vi "GetErrorLog.vi"(6 "Delay between send and receive [ms]":i32=100, 8 "error in (no error)":errorcluster, 11 "SCD in":refnum<class "SCD.lvclass">) -> (0 "error out":errorcluster, 1 "Found?":bool, 2 "errors":string[](array[string]), 3 "SCD out":refnum<class "SCD.lvclass">)   [LabVIEW 2023, in "horiba.lvlib" / "SCD.lvclass"]
doc: "Gets the integration time that was previously set. If no integration time has been explicitly set, the default value is returned.\nThe integration time is returned in seconds."
uses:
  SCD.lvclass
  b6349250-cb33-415b-847a-a7f5d99734f6.vi
  <vilib>/JDP Science/JSONtext/Variant to JSON Text.vi
  <vilib>/JDP Science/JSONtext/Set Item.vi
  <vilib>/JDP Science/JSONtext/JSON text to Variant.vi
  <vilib>/JDP Science/JSONtext/LVClass Serializer/JSONtext LVClass Serializer.lvclass
  SCD.lvclass/SCD.ctl
  GenericDevice/GenericDevice.lvclass
  77142ea6-4bc9-4026-b9b5-fb5d7ddf8a7e.vi
panel:
  # "Connector Pane"
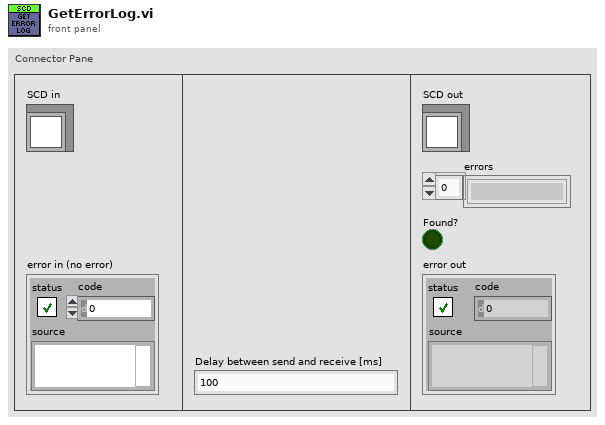
[diagram p1: front panel]
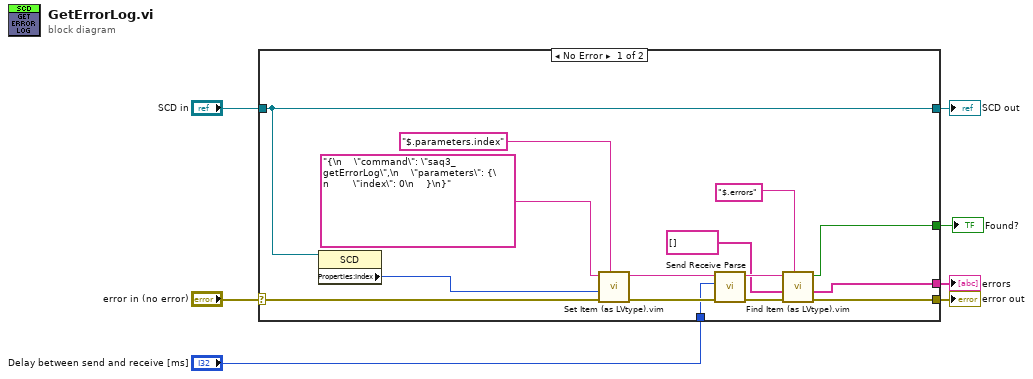
[diagram p0: block diagram]
diagram:
  n1 = case shown="No Error" "error in (no error)" {
    selector: "error in (no error)" -> [w18 w24]
    tunnel: [w11 w24] -> w3
    tunnel: [w20 w23] -> w5
    tunnel: "SCD in" -> [w20 w23]
    tunnel: "Delay between send and receive [ms]" -> [w15 _]
    tunnel: [w9 _] -> w2
    tunnel: [w8 _] -> w1
    frame No Error {
      n2 = property class="SCD"(reference=w20) -> ("Properties:Index"=w19:i32)  [unwired: 1 in, 2 out]
      n3 = call "Set Item (as LVtype).vim"("$Path or Item Name"="$.parameters.index", "error in (no error)"=w18, "Anything"=w19, "JSON"="{\n    \"command\": \"saq3_getErrorLog\",\n    \"parameters\": {\n        \"index\": 0\n    }\n}") -> ("error out"=w16:errorcluster, "<JSON>"=w14:string)  [unwired: 4 in, 1 out]
      n4 = call "Send Receive Parse.vi"("error in"=w16, "Delay between send and receive [ms]"=w15, "<JSON>"=w14) -> ("error out"=w12:errorcluster, "results-JSON string"=w17:string)  [unwired: 6 in, 1 out]
      n5 = call "Find Item (as LVtype).vim"("$Path or Item Name"="$.errors", "error in (no error)"=w12, "Data Type and Default Value"=string[] [] ("errors"), "JSON"=w17) -> ("error out"=w11:errorcluster, "Data"=w9:string[], "Found"=w8:bool)  [unwired: 4 in, 1 out]
    }
    frame Error {
    }
  }
  "error out" <- w3
  "SCD out" <- w5
  "errors" <- w2
  "Found?" <- w1
